vi "Get Data.vi"(8 "error in (no error)":errorcluster, 11 "Xitron in":refnum<class "Xitron.lvclass">) -> (0 "error out":errorcluster, 2 "Data Out":T1[](array[typedef]), 3 "Xitron out":refnum<class "Xitron.lvclass">)   [LabVIEW 2015, in "Xitron.lvclass"]
uses:
  Xitron.lvclass
  Parent/Power Data.ctl
  Parent/Power Meter.lvclass/Power Meter.ctl
  Parent/Read Address.vi
  Parent/Power Meter.lvclass
panel:
  out "DataStr":string
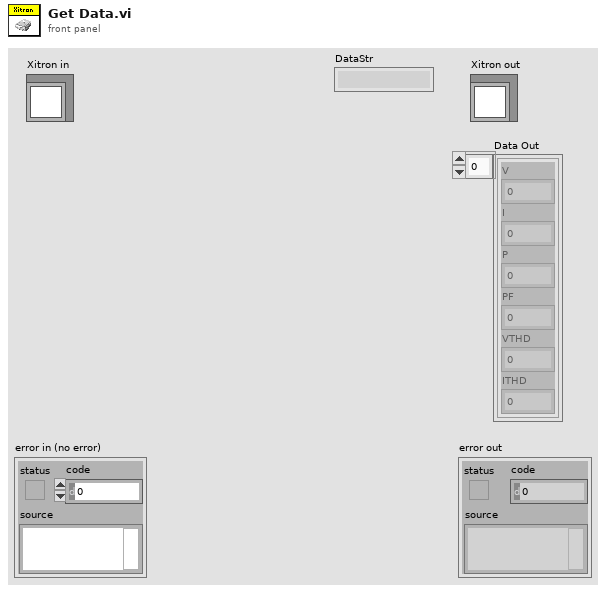
[diagram p1: front panel]
types:
  T1 = typedef "Power Meter.lvclass/Power Data.ctl" = cluster{"V":dbl, "I":dbl, "P":dbl, "PF":dbl, "VTHD":dbl, "ITHD":dbl}
  T2 = cluster{"[0]":dbl, "[1]":dbl, "[2]":dbl, "[3]":dbl, "[4]":dbl, "[5]":dbl}
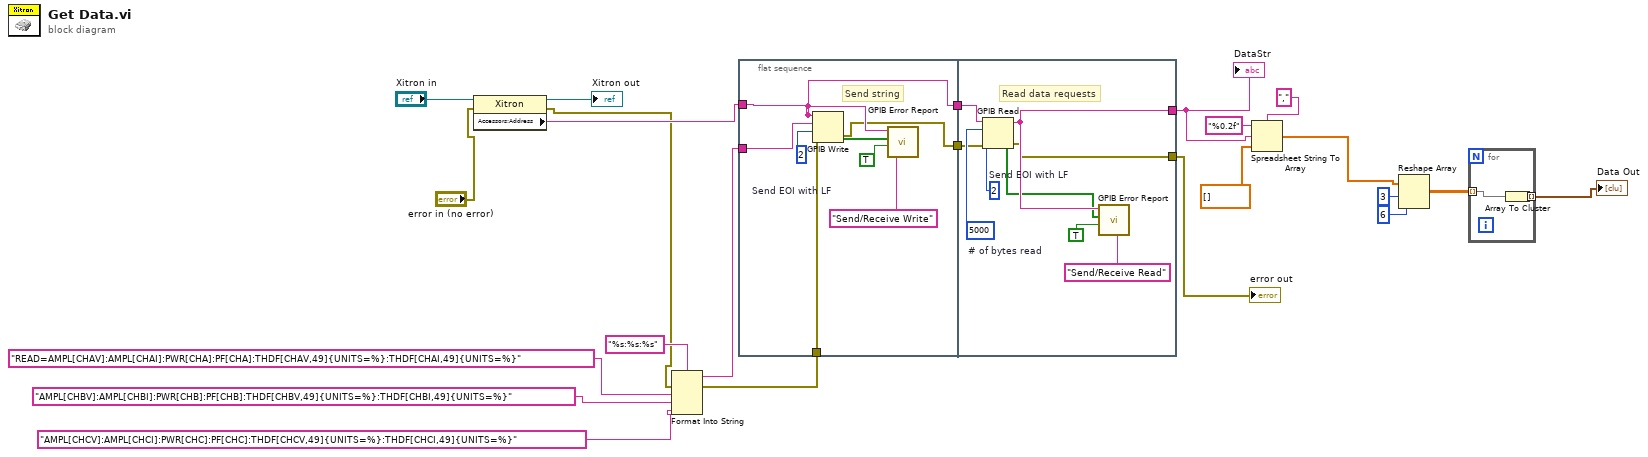
[diagram p0: block diagram]
diagram:
  n1 = property class="Xitron"(reference="Xitron in", error in="error in (no error)") -> (reference out=→"Xitron out":refnum<class "Xitron.lvclass">, error out=w9:errorcluster, "Accessors:Address"=w20:string)
  n2 = Format Into String(format string="%s:%s:%s", error in=w9, "READ=AMPL[CHAV]:AMPL[CHAI]:PWR[CHA]:PF[CHA]:THDF[CHAV,49]{UNITS=%}:THDF[CHAI,49]{UNITS=%}", "AMPL[CHBV]:AMPL[CHBI]:PWR[CHB]:PF[CHB]:THDF[CHBV,49]{UNITS=%}:THDF[CHBI,49]{UNITS=%}", "AMPL[CHCV]:AMPL[CHCI]:PWR[CHC]:PF[CHC]:THDF[CHCV,49]{UNITS=%}:THDF[CHCI,49]{UNITS=%}") -> (resulting string=w13:string, error out=w8:errorcluster)  [unwired: 1 in]
  n3 = flat-sequence {
    tunnel: [w26] -> w23
    tunnel: w13 -> [w30]
    tunnel: w20 -> [w26]
    tunnel: w8 -> [w25]
    tunnel: [w24] -> w7
    tunnel: w23 -> [w38]
    tunnel: [w37] -> w12
    tunnel: w7 -> [w33]
    tunnel: [w32] -> w6
    frame #0 {
      w31 = 2  # Send EOI with LF
      # "Send string"
      n4 = GPIB Write(0:w26, 1:w30, 2:w31, 3:w25) -> (5:w29:bool[], 6:w24:errorcluster)  [unwired: 1 in]
      n5 = call "GPIB Error Report.vi"("Function"="Send/Receive Write", "Dialog?(F)"=TRUE, "Status"=w29, "Address String"=w26) -> ()  [unwired: 2 out]
    }
    frame #1 {
      w39 = 5000  # # of bytes read
      w40 = 2  # Send EOI with LF
      # "Read data requests"
      n6 = GPIB Read(0:w38, 1:w39, 2:w40, 3:w33) -> (5:w37:string, 6:w36:bool[], 7:w32:errorcluster)  [unwired: 1 in]
      n7 = call "GPIB Error Report.vi"("Function"="Send/Receive Read", "Dialog?(F)"=TRUE, "Status"=w36, "Address String"=w37) -> ()  [unwired: 2 out]
    }
  }
  n8 = Spreadsheet String To Array(delimiter (Tab)=",", format string="%0.2f", spreadsheet string=w12, array type (2D Dbl)=dbl[] []) -> (array=w5:dbl[])
  n9 = Reshape Array(w5, 3 ("dimension size"), 6 ("dimension size")) -> (w2:dbl[][])
  n10 = for {
    tunnel: w2 -> [w42] mode=indexing
    tunnel: [w41] -> w1 mode=indexing
    n11 = Array To Cluster(array=w42) -> (cluster=w41:T2)
  }
  "Data Out" <- w1
  "error out" <- w6
  "DataStr" <- w12
